vi "Facade.vi"(0 "Data In":T4, 2 "Display State In":T2, 3 "Container State":T3) -> (6 "Data Out":T4, 7 "Display State Out":T2, 8 "Action":T1)   [LabVIEW 2011, in "High Light Button.xctl"]
doc: "Reference:\nhttp://ruanqizhen.spaces.live.com/blog/cns!5852D4F797C53FB6!1973.entry"
uses:
  High Light Button.xctl
  Data.ctl
  <vilib>/_xctls/Container State.ctl
  State.ctl
  <vilib>/_xctls/Action.ctl
  <vilib>/_xctls/XControlSupport.lvlib
panel:
  in  "data":bool
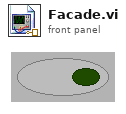
[diagram p1: front panel]
types:
  T1 = typedef "XControlSupport.lvlib/Action.ctl" = cluster{"Data Changed?":bool, "State Changed?":bool, "Action Name":string}
  T2 = typedef "High Light Button.xctl/State.ctl" = cluster{"Numeric":dbl}
  T3 = typedef "XControlSupport.lvlib/Container State.ctl" = cluster{"Indicator?":bool, "Run Mode?":bool, " Refnum":refnum<vi>}
  T4 = typedef "High Light Button.xctl/Data.ctl" = bool
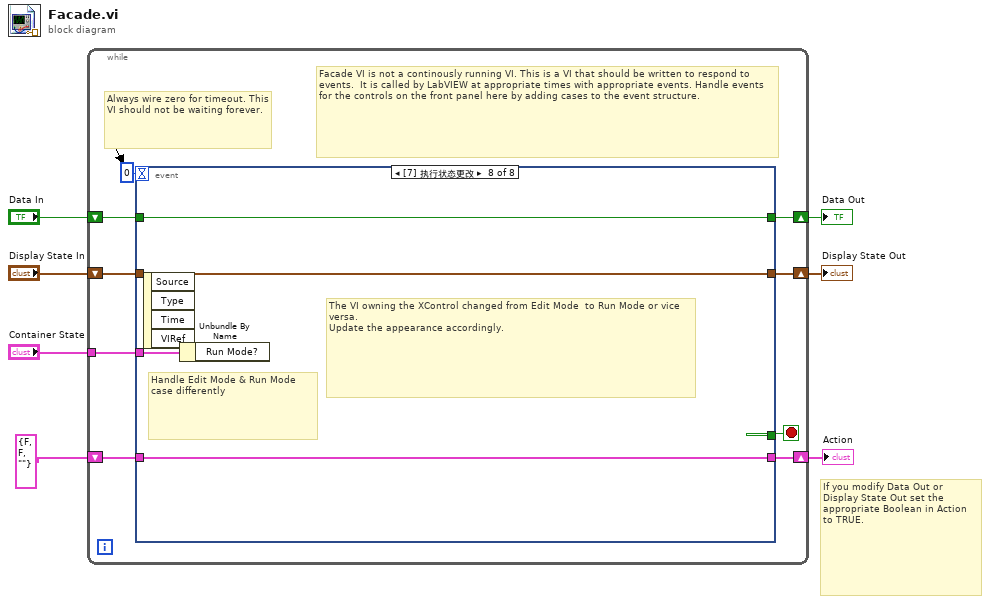
[diagram p0: block diagram]
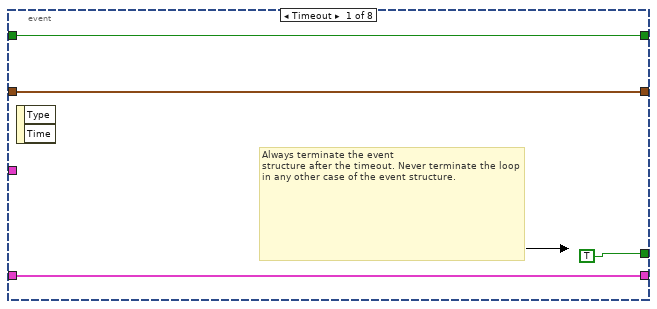
[diagram p2: hidden frame]
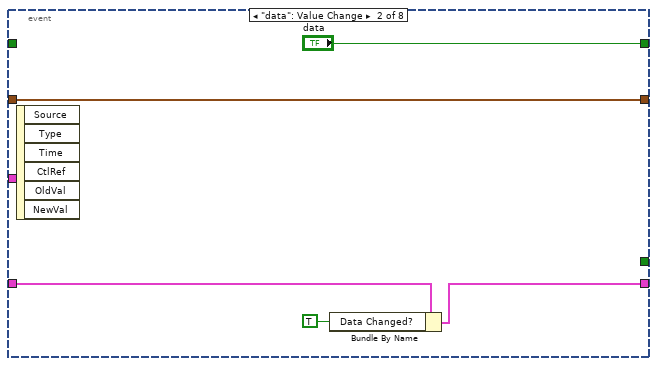
[diagram p3: hidden frame]
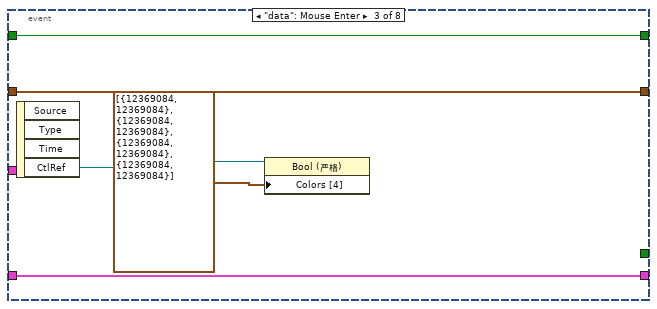
[diagram p4: hidden frame]
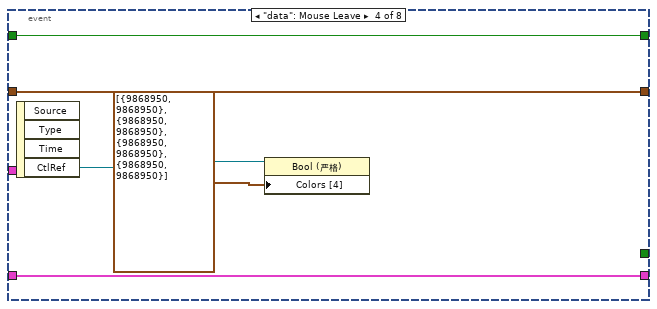
[diagram p5: hidden frame]
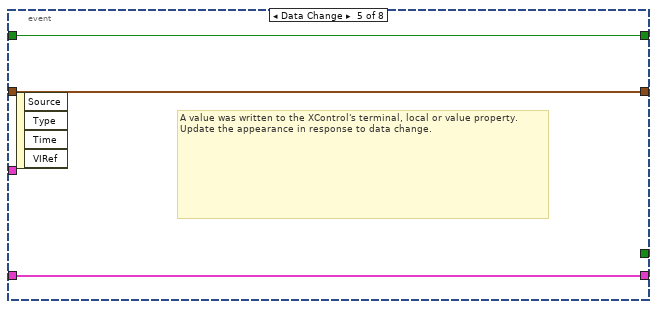
[diagram p6: hidden frame]
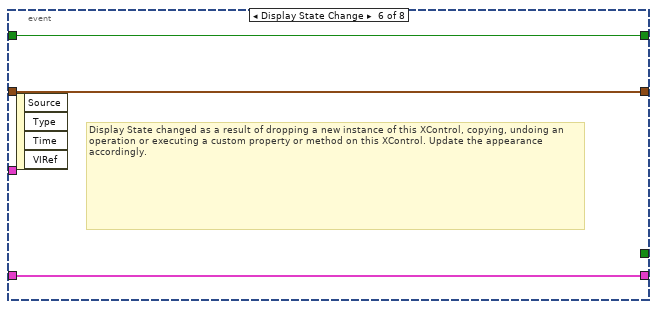
[diagram p7: hidden frame]
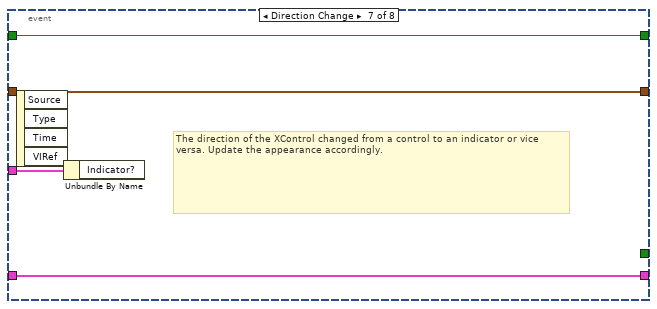
[diagram p8: hidden frame]
diagram:
  # "If you modify Data Out or\nDisplay State Out set the\nappropriate Boolean in Action\nto TRUE."
  n1 = while {
    shift-right: [w15] -> w4
    shift-left: "Display State In" -> [w16]
    tunnel: "Container State" -> [w12]
    shift-right: [w10] -> w7
    shift-left: "Data In" -> [w11]
    shift-right: [w8] -> w2
    shift-left: T1 {"Data Changed?"=FALSE, "State Changed?"=FALSE, "Action Name"=""} ("Action") -> [w9]
    stop <- w14 stop-if-true
    # "Facade VI is not a continously running VI. This is a VI that should be written to respond to events.  It is called by LabVIEW at appropriate times with appropriate events. Handle events for the controls on the front panel here by adding cases to the event structure."
    # "Always wire zero for timeout. This\nVI should not be waiting forever."
    n2 = event shown="[7] 执行状态更改" {
      selector: _ -> [_ _ _ _ _ _ _ _]
      dyn-events: _ -> [_ _ _ _ _ _ _ _]
      timeout: 0 -> [_ _ _ _ _ _ _ _]
      tunnel: w16 -> [w19 w24 w28 w32 w37 w41 w44 w48]
      tunnel: [w19 w24 w28 w32 w37 w41 w44 w48] -> w15
      tunnel: [TRUE _ _ _ _ _ _ _] -> w14
      tunnel: w12 -> [_ _ _ _ _ _ w45 w49]
      tunnel: w11 -> [w18 _ w27 w33 w38 w40 w43 w47]
      tunnel: [w18 "data" w27 w33 w38 w40 w43 w47] -> w10
      tunnel: [w17 w21 w26 w31 w36 w39 w42 w46] -> w8
      tunnel: w9 -> [w17 w23 w26 w31 w36 w39 w42 w46]
      event Timeout {
        # "Always terminate the event\nstructure after the timeout. Never terminate the loop in any other case of the event structure."
        n3 = event-data() -> ()  [unwired: 1 in, 2 out]
      }
      event "data": Value Change {
        n4 = event-data() -> ()  [unwired: 1 in, 6 out]
        n5 = Bundle By Name(cluster=w23, "Data Changed?"=TRUE) -> (w21:T1)
      }
      event "data": Mouse Enter {
        n6 = event-data() -> ("CtlRef"=w30:refnum<vi>)  [unwired: 1 in, 3 out]
        n7 = property class="Bool (严格)"(reference=w30, "Colors [4]"=cluster{u32, u32}[] [{12369084, 12369084}, {12369084, 12369084}, {12369084, 12369084}, {12369084, 12369084}]) -> ()  [unwired: 1 in, 2 out]
      }
      event "data": Mouse Leave {
        n8 = event-data() -> ("CtlRef"=w35:refnum<vi>)  [unwired: 1 in, 3 out]
        n9 = property class="Bool (严格)"(reference=w35, "Colors [4]"=cluster{u32, u32}[] [{9868950, 9868950}, {9868950, 9868950}, {9868950, 9868950}, {9868950, 9868950}]) -> ()  [unwired: 1 in, 2 out]
      }
      event Data Change {
        # "A value was written to the XControl's terminal, local or value property.\nUpdate the appearance in response to data change."
        n10 = event-data() -> ()  [unwired: 1 in, 4 out]
      }
      event Display State Change {
        # "Display State changed as a result of dropping a new instance of this XControl, copying, undoing an operation or executing a custom property or method on this XControl. Update the appearance accordingly."
        n11 = event-data() -> ()  [unwired: 1 in, 4 out]
      }
      event Direction Change {
        # "The direction of the XControl changed from a control to an indicator or vice versa. Update the appearance accordingly."
        n12 = event-data() -> ()  [unwired: 1 in, 4 out]
        n13 = Unbundle By Name(w45) -> ()  [unwired: 1 out]
      }
      event Exec State Change {
        # "The VI owning the XControl changed from Edit Mode  to Run Mode or vice versa.\nUpdate the appearance accordingly."
        # "Handle Edit Mode & Run Mode\ncase differently"
        n14 = event-data() -> ()  [unwired: 1 in, 4 out]
        n15 = Unbundle By Name(w49) -> ()  [unwired: 1 out]
      }
    }
  }
  "Display State Out" <- w4
  "Data Out" <- w7
  "Action" <- w2
